vi "New Focus - rétroaction.vi"() -> ()   [LabVIEW 2017]
uses:
  dll/CmdLib.dll
  Type Def/Data cluster.ctl
panel:
  in  "Wavelength (nm)":u32=1064
  in  "Pas":i32=10
  in  "angle du max":i32=4500
  in  "ParameterPhi":dbl=38.36882237534376
  in  "ParameterC":dbl=2.6797703442087277
  in  "ParameterB":dbl=1.035346678618637e-36
  in  "ParameterA":dbl=0.997938844220231
  out "nombre":dbl
  out "DAQ?":bool
  in  "Mode":bool
  in  "VISA Refnum in":refnum<visa-resource-name>
  in  "consigne":dbl=23.0 format="%#_13g"
  in  "erreur en %":dbl(knob)=2.0 scale=0.0..10.0
  in  "Bouton Piste suivante":bool
  in  "Bouton Recherche en avant":bool
  in  "Bouton Recherche en arrière":bool
  in  "Bouton Piste précédente":bool
  out "tampon":i32=50
  out "Taux transmission calculé":dbl
  in  "Taux Transmission":dbl(knob)=0.98 min=0.02 max=0.98 scale=0.0..1.0
  in  "Maximum?":bool
  in  "Relative Steps":i32=50
  out "sortie d'erreur":errorcluster
  in  "Motor 3":bool
  in  "Motor 2":bool
  in  "Motor 1":bool
  in  "Bouton Stop":bool
  out "DeviceKey List Out":string[](array[string])
  out "error IO":errorcluster
  out "error out":errorcluster
  out "Device Array":T1(array[cluster])
  out "CmdLib Out":refnum<k24>
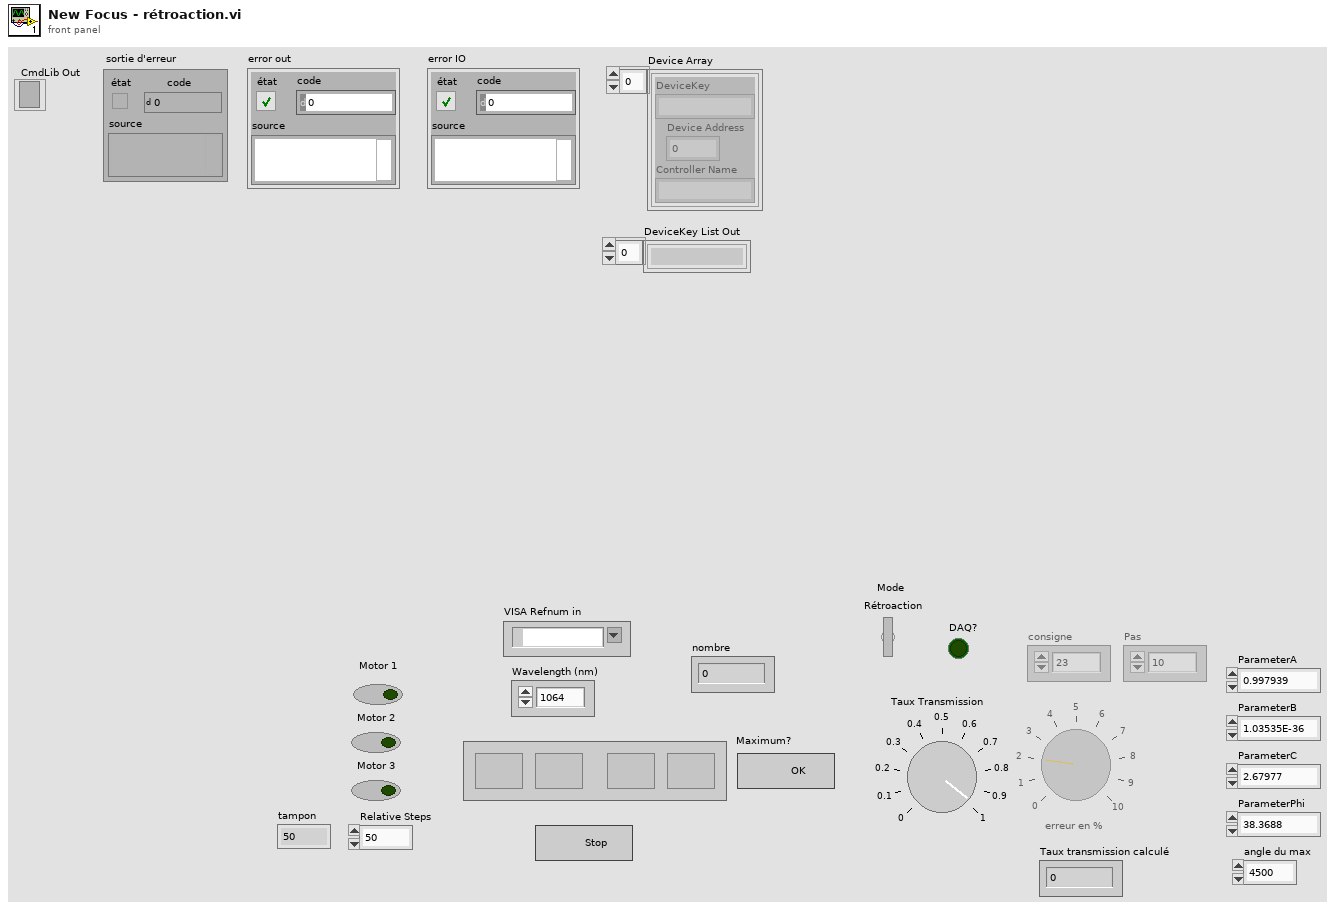
[diagram p1: front panel]
types:
  T1 = cluster{"DeviceKey":string, "Device Address":i32, "Controller Name":string}[]
  T2 = enum8{"Enabled", "Disabled", "Disabled and Grayed Out"}
  T3 = typedef "Data cluster.ctl" = cluster{enum16{"Init", "Control", "Stop"}, "Device Adress":i32, "Motor":i32, "Device Key":string, "Relative Steps":i32}
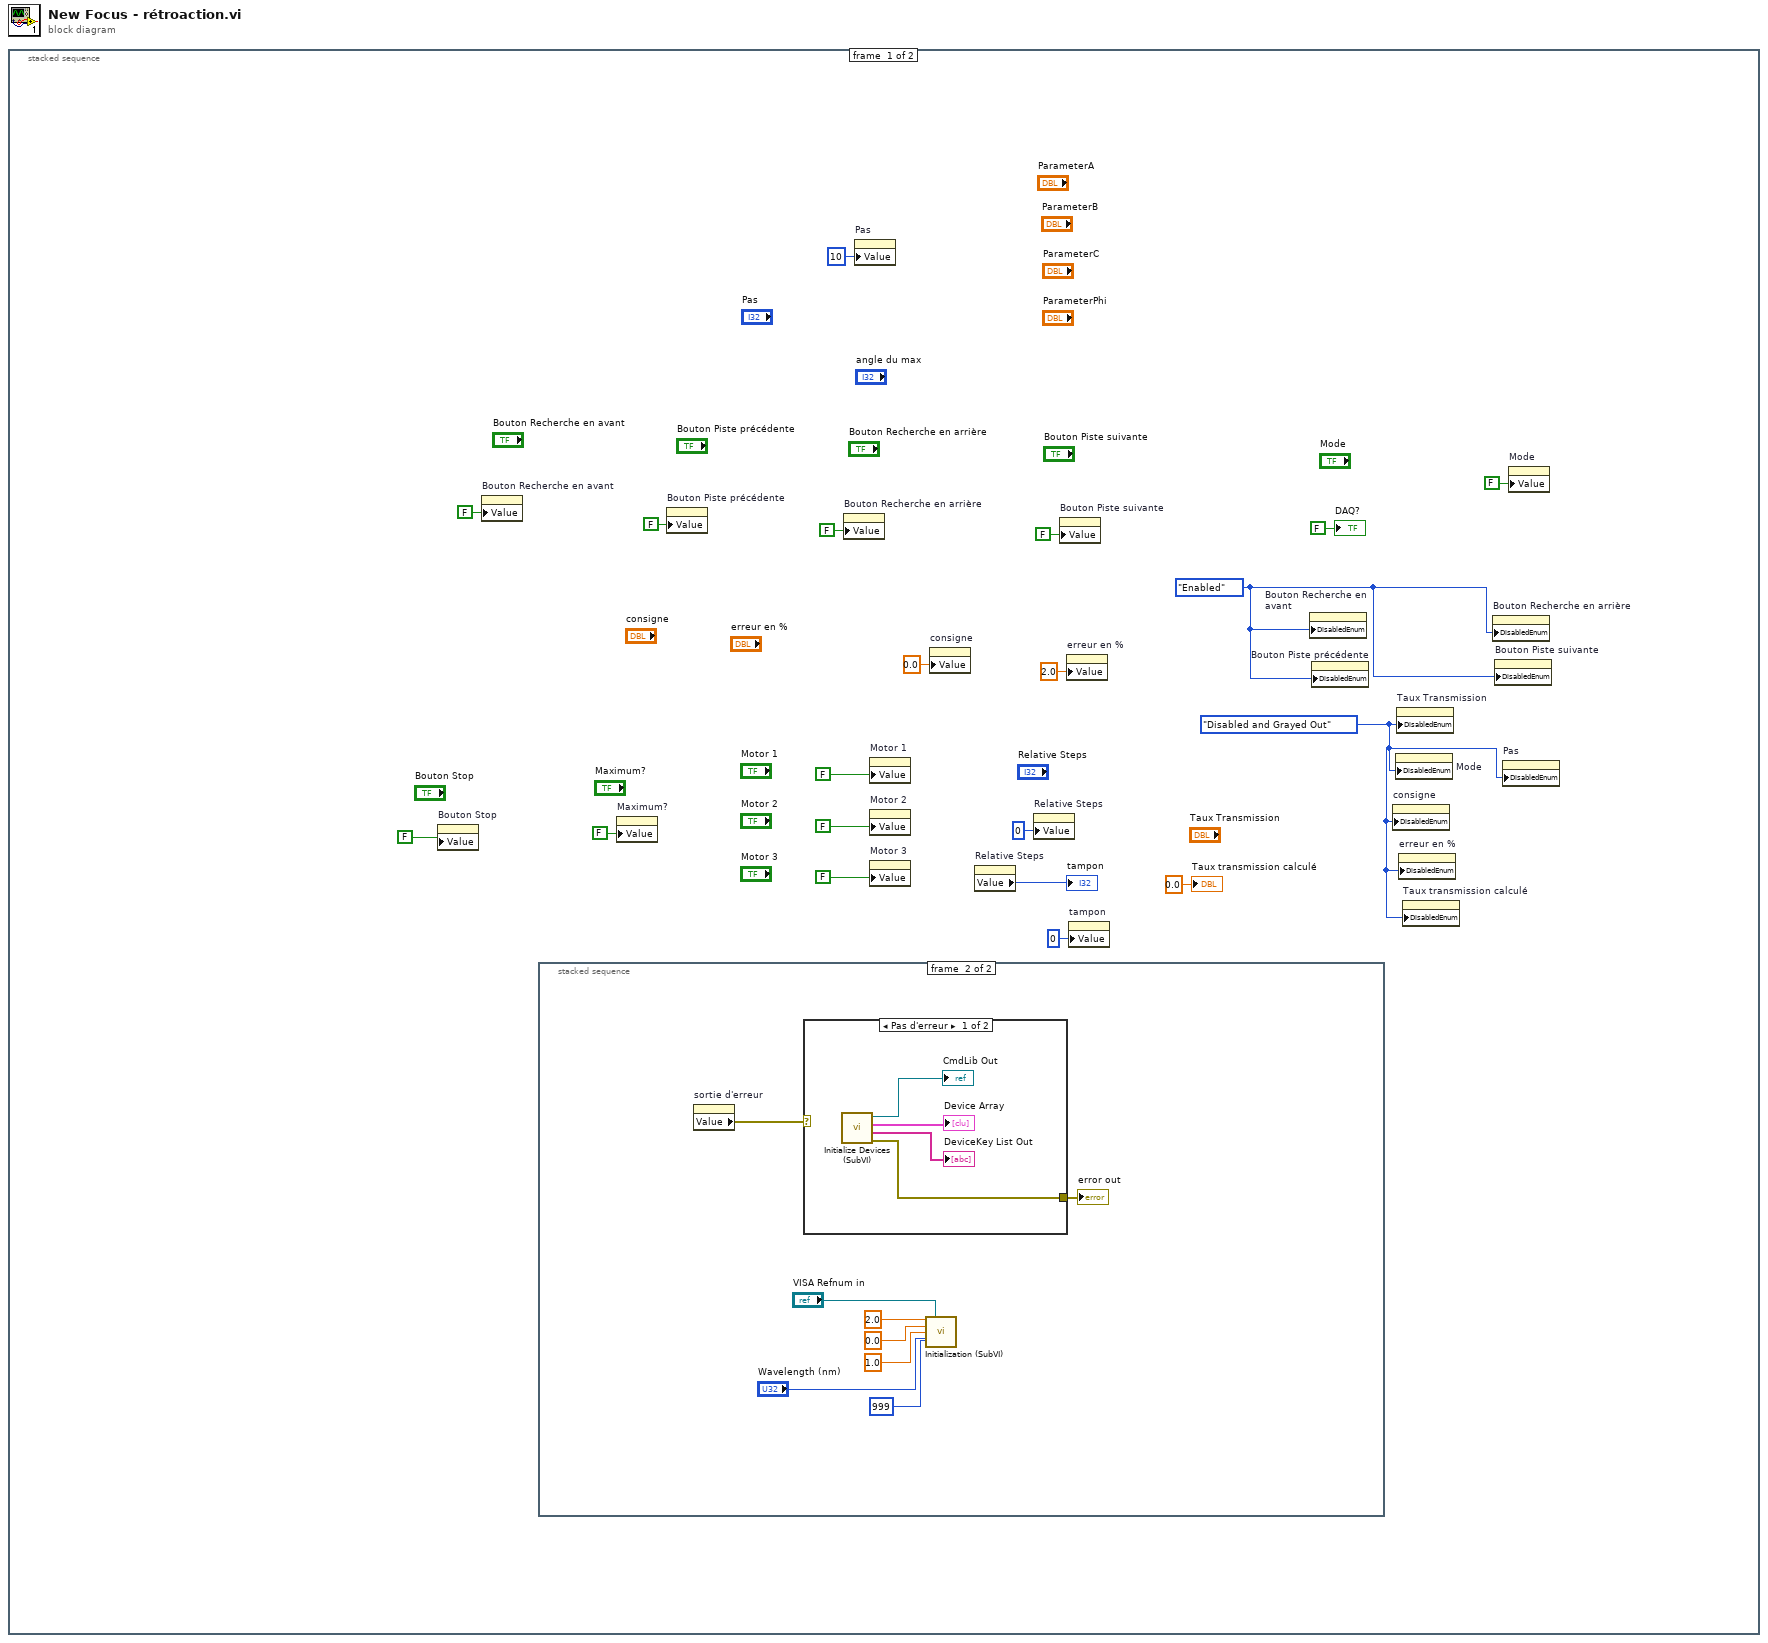
[diagram p0: block diagram]
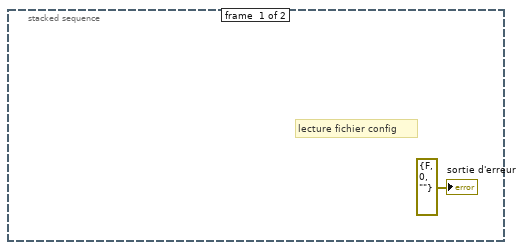
[diagram p2: hidden frame]
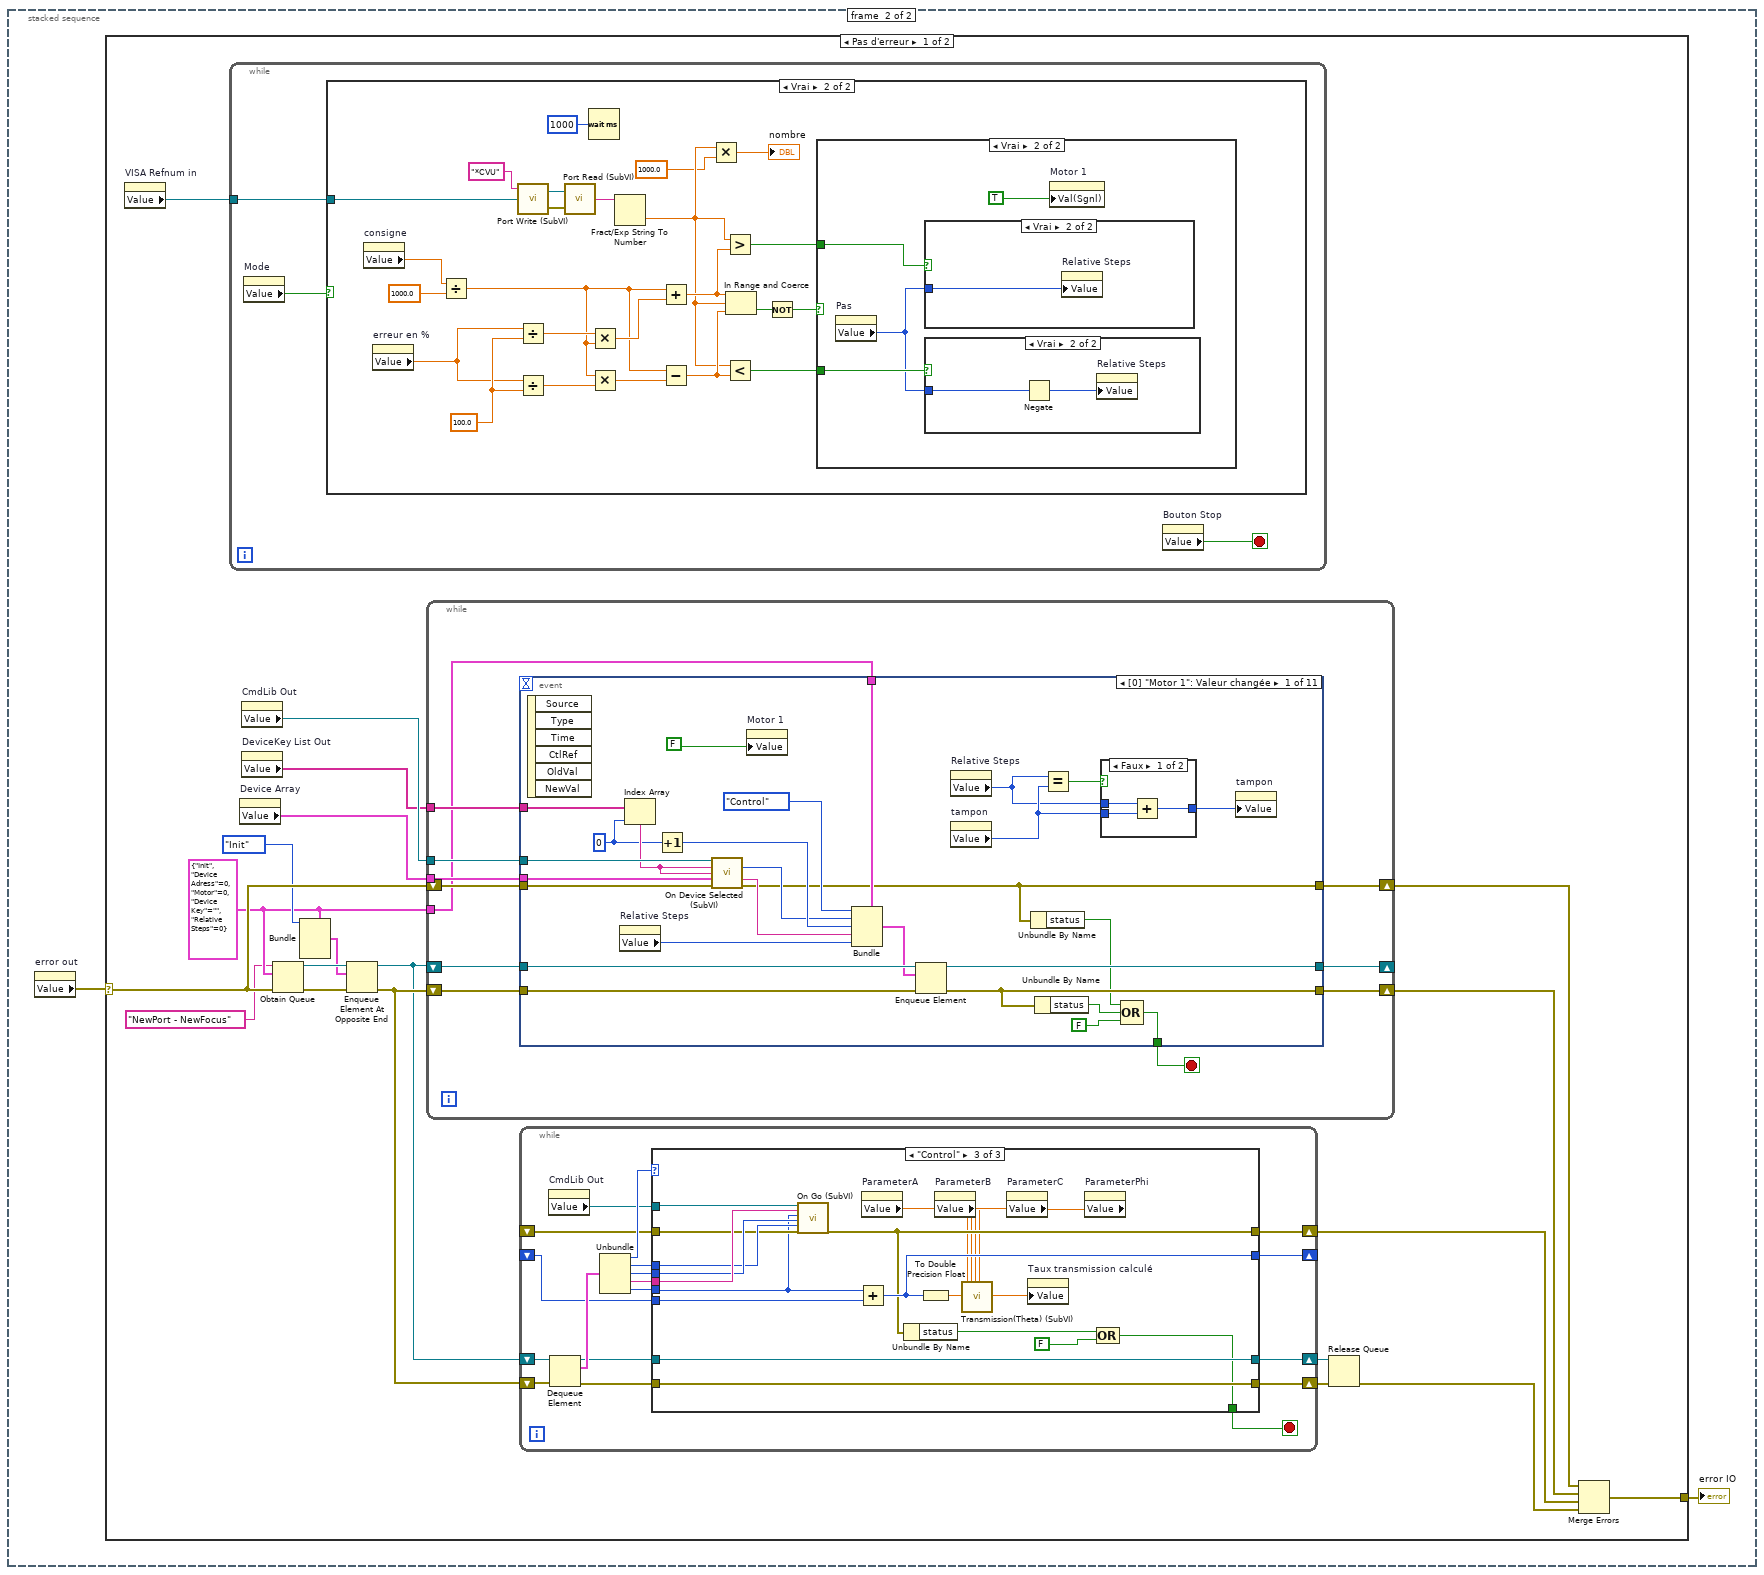
[diagram p4: hidden frame]
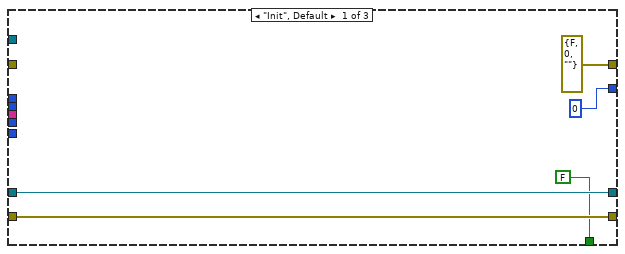
[diagram p9: hidden frame]
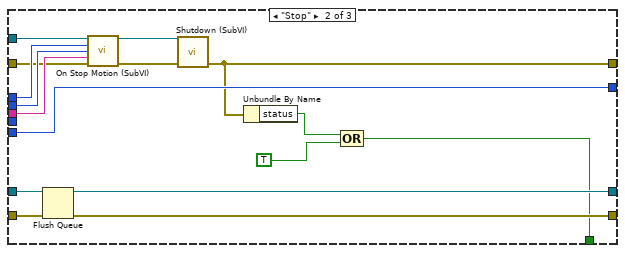
[diagram p10: hidden frame]
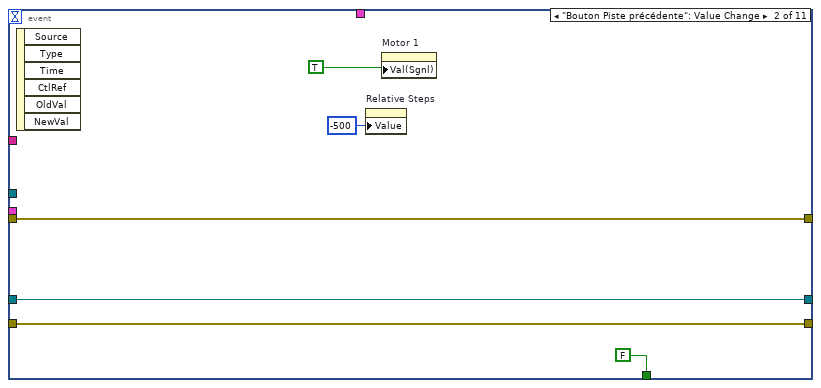
[diagram p12: hidden frame]
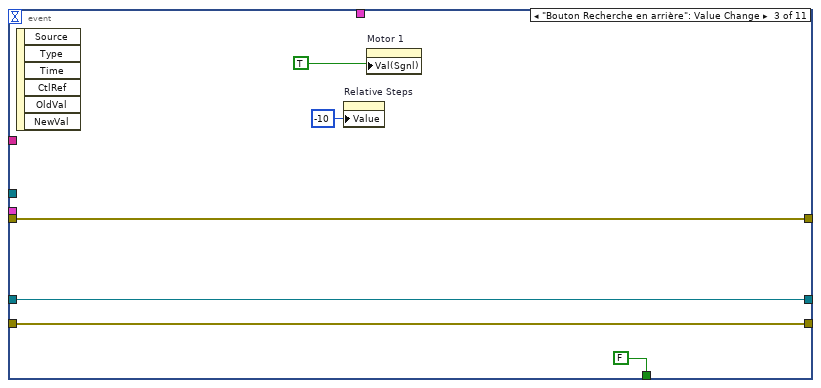
[diagram p13: hidden frame]
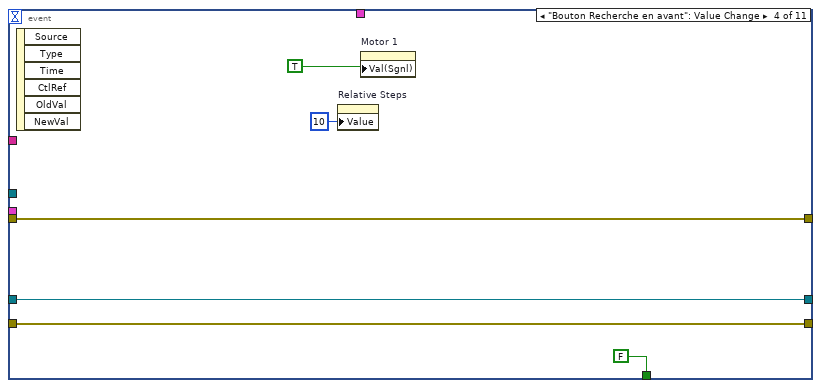
[diagram p14: hidden frame]
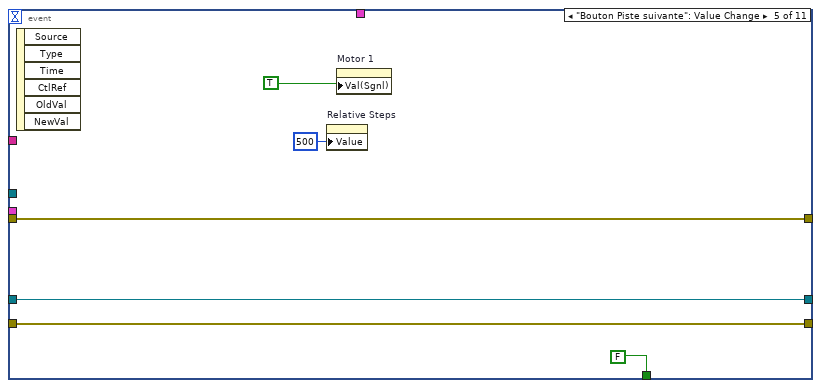
[diagram p15: hidden frame]
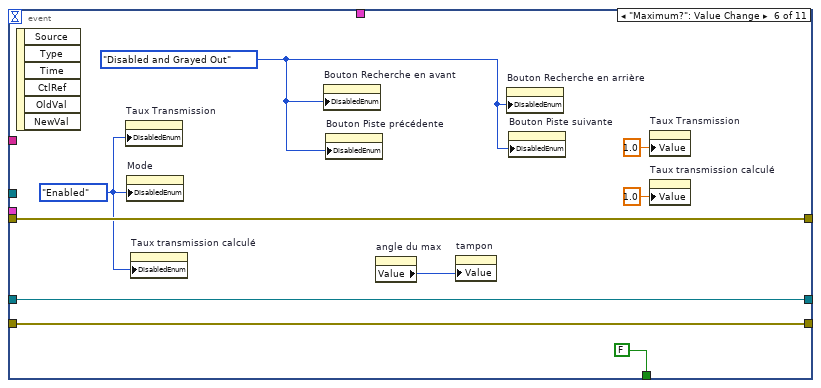
[diagram p16: hidden frame]
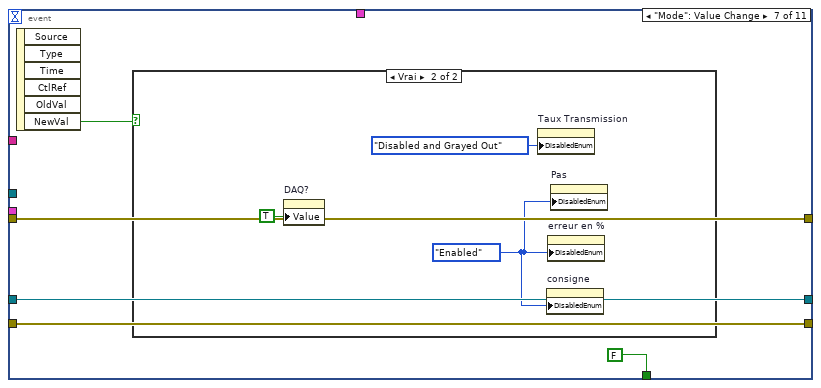
[diagram p17: hidden frame]
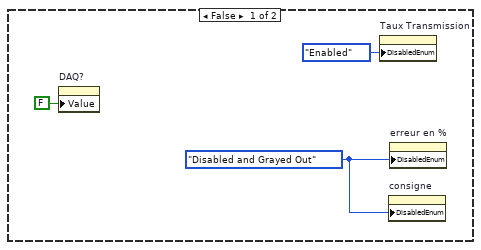
[diagram p18: hidden frame]
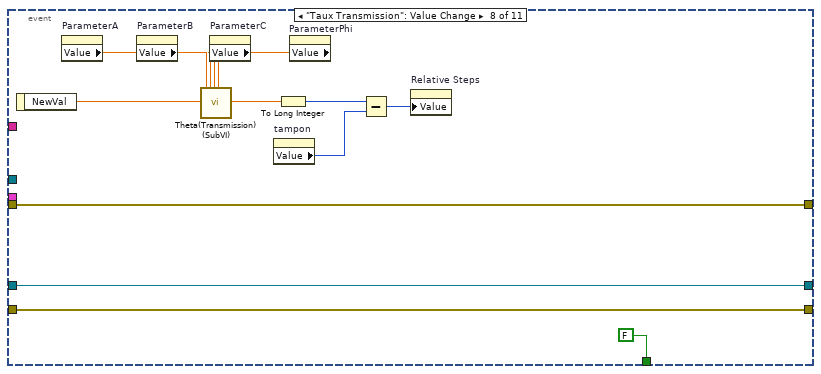
[diagram p19: hidden frame]
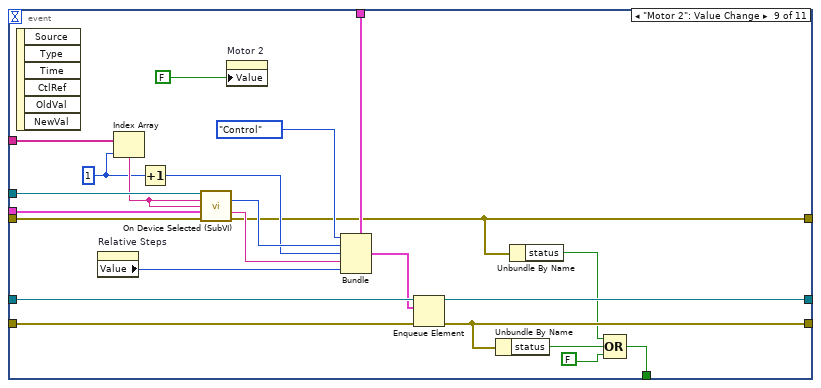
[diagram p20: hidden frame]
diagram:
  n1 = stacked-sequence {
    frame #0 {
      w2 = T2."Disabled and Grayed Out" ("Désactivé")
      w8 = T2."Enabled" ("Désactivé")
      n2 = property on="Bouton Stop" class="Bool (strict)"("Value"=FALSE) -> ()  [unwired: 2 in, 2 out]
      n3 = property on="Bouton Recherche en avant" class="Bool (strict)"("Value"=FALSE ("Bouton Recherche en avant")) -> ()  [unwired: 2 in, 2 out]
      n4 = stacked-sequence {
        frame #0 {
          # "lecture fichier config"
          "sortie d'erreur" <- errorcluster {"status"=FALSE, "code"=0, "source"=""} ("sortie d'erreur")
        }
        frame #1 {
          n5 = property on="sortie d'erreur" class="Clust (strict)"() -> ("Value"=w28:errorcluster)  [unwired: 2 in, 2 out]
          n6 = case shown="Pas d'erreur" w28 {
            selector: w28 -> [_ w34]
            tunnel: [w33 w34] -> w29
            frame No Error {
              n7 = call "Initialize Devices (SubVI).vi"() -> ("sortie d'erreur"=w33:errorcluster, "DeviceKey List Out"=→"DeviceKey List Out":string[], "Device Array"=→"Device Array":T1, "Refnum de .NET en sortie"=→"CmdLib Out":refnum<k24>)  [unwired: 8 in]
            }
            frame Error {
            }
          }
          "error out" <- w29
          n8 = call "Initialization (SubVI).vi"("Trigger Level (% of Scale)"=2.0, "VISA Refnum in"="VISA Refnum in", "Offset"=sgl 0.0, "Multiplier"=sgl 1.0, "Wavelength (nm)"="Wavelength (nm)", "Scale"=u32 999) -> ()  [unwired: 8 in, 2 out]
        }
      }
      n9 = property on="Maximum?" class="Bool (strict)"("Value"=FALSE ("Minimum?")) -> ()  [unwired: 2 in, 2 out]
      n10 = property on="Bouton Piste précédente" class="Bool (strict)"("Value"=FALSE ("Bouton Piste précédente")) -> ()  [unwired: 2 in, 2 out]
      n11 = property on="Bouton Recherche en arrière" class="Bool (strict)"("Value"=FALSE ("Bouton Recherche en arrière")) -> ()  [unwired: 2 in, 2 out]
      n12 = property on="Pas" class="NumNb (strict)"("Value"=10 ("Numérique")) -> ()  [unwired: 2 in, 2 out]
      n13 = property on="Motor 1" class="Bool (strict)"("Value"=FALSE) -> ()  [unwired: 2 in, 2 out]
      n14 = property on="Motor 2" class="Bool (strict)"("Value"=FALSE) -> ()  [unwired: 2 in, 2 out]
      n15 = property on="Motor 3" class="Bool (strict)"("Value"=FALSE) -> ()  [unwired: 2 in, 2 out]
      n16 = property on="consigne" class="NumNb (strict)"("Value"=0.0 ("consigne")) -> ()  [unwired: 2 in, 2 out]
      n17 = property on="Relative Steps" class="NumNb (strict)"() -> ("Value"=→"tampon":i32)  [unwired: 2 in, 2 out]
      n18 = property on="Relative Steps" class="NumNb (strict)"("Value"=0 ("Relative Steps")) -> ()  [unwired: 2 in, 2 out]
      n19 = property on="Bouton Piste suivante" class="Bool (strict)"("Value"=FALSE ("Bouton Piste suivante")) -> ()  [unwired: 2 in, 2 out]
      n20 = property on="erreur en %" class="BoutRot (strict)"("Value"=2.0 ("erreur en %")) -> ()  [unwired: 2 in, 2 out]
      n21 = property on="tampon" class="NumNb (strict)"("Value"=0 ("tampon")) -> ()  [unwired: 2 in, 2 out]
      n22 = property on="Bouton Recherche en avant" class="Bool (strict)"("DisabledEnum"=w8) -> ()  [unwired: 2 in, 2 out]
      n23 = property on="Bouton Piste précédente" class="Bool (strict)"("DisabledEnum"=w8) -> ()  [unwired: 2 in, 2 out]
      n24 = property on="consigne" class="NumNb (strict)"("DisabledEnum"=w2) -> ()  [unwired: 2 in, 2 out]
      n25 = property on="Mode" class="Bool (strict)"("DisabledEnum"=w2) -> ()  [unwired: 2 in, 2 out]
      n26 = property on="Taux Transmission" class="BoutRot (strict)"("DisabledEnum"=w2) -> ()  [unwired: 2 in, 2 out]
      n27 = property on="erreur en %" class="BoutRot (strict)"("DisabledEnum"=w2) -> ()  [unwired: 2 in, 2 out]
      n28 = property on="Taux transmission calculé" class="NumNb (strict)"("DisabledEnum"=w2) -> ()  [unwired: 2 in, 2 out]
      n29 = property on="Bouton Recherche en arrière" class="Bool (strict)"("DisabledEnum"=w8) -> ()  [unwired: 2 in, 2 out]
      n30 = property on="Bouton Piste suivante" class="Bool (strict)"("DisabledEnum"=w8) -> ()  [unwired: 2 in, 2 out]
      n31 = property on="Pas" class="NumNb (strict)"("DisabledEnum"=w2) -> ()  [unwired: 2 in, 2 out]
      n32 = property on="Mode" class="Bool (strict)"("Value"=FALSE ("Mode")) -> ()  [unwired: 2 in, 2 out]
      "Taux transmission calculé" <- 0.0 ("x-y")
      "DAQ?" <- FALSE ("DAQ?")
    }
    frame #1 {
      n33 = property on="error out" class="Clust (strict)"() -> ("Value"=w36:errorcluster)  [unwired: 2 in, 2 out]
      n34 = case shown="Pas d'erreur" w36 {
        selector: w36 -> [w55 w327]
        tunnel: [w56 w327] -> w35
        frame No Error {
          w48 = T3 {enum."Init", "Device Adress"=0, "Motor"=0, "Device Key"="", "Relative Steps"=0}
          n35 = property on="VISA Refnum in" class="NomVISA"() -> ("Value"=w37:refnum<visa-resource-name>)  [unwired: 2 in, 2 out]
          n36 = while {
            tunnel: w37 -> [w57]
            stop <- w59 stop-if-true
            n37 = property on="Mode" class="Bool (strict)"() -> ("Value"=w58:bool)  [unwired: 2 in, 2 out]
            n38 = case shown="Vrai" w58 {
              tunnel: w57 -> [_ w66]
              frame False {
              }
              frame True {
                w74 = 100.0 ("y")
                n39 = property on="consigne" class="NumNb (strict)"() -> ("Value"=w61:dbl)  [unwired: 2 in, 2 out]
                n40 = property on="erreur en %" class="BoutRot (strict)"() -> ("Value"=w71:dbl)  [unwired: 2 in, 2 out]
                n41 = Divide(x=w61, y=1000.0) -> (x/y=w62:dbl)
                n42 = call "Port Write (SubVI).vi"("VISA Refnum in"=w66, "write buffer"="*CVU") -> ("error out"=w80:errorcluster, "VISA Refnum out"=w81:refnum<visa-resource-name>)  [unwired: 1 in]
                n43 = Divide(x=w71, y=w74) -> (x/y=w78:dbl)
                n44 = Divide(x=w71, y=w74) -> (x/y=w75:dbl)
                n45 = call "Port Read (SubVI).vi"("VISA Refnum in"=w81, "error in"=w80) -> ("buffer read"=w79:string)  [unwired: 2 out]
                n46 = Wait (ms)(milliseconds to wait=u32 1000 ("attente (ms)")) -> ()  [unwired: 1 out]
                n47 = Multiply(x=w78, y=w62) -> (x*y=w76:dbl)
                n48 = Multiply(x=w62, y=w75) -> (x*y=w77:dbl)
                n49 = Fract/Exp String To Number(string=w79) -> (number=w64:dbl)  [unwired: 3 in, 1 out]
                n50 = Add(x=w62, y=w76) -> (x+y=w73:dbl)
                n51 = Subtract(x=w62, y=w77) -> (x-y=w72:dbl)
                n52 = Multiply(x=w64, y=1000.0) -> (x*y=→"nombre":dbl)
                n53 = Greater?(x=w64, y=w73) -> (0:w69:bool)
                n54 = Less?(x=w64, y=w72) -> (x < y?=w70:bool)
                n55 = In Range and Coerce(upper limit=w73, x=w64, lower limit=w72) -> (In Range?=w68:bool)  [unwired: 1 out]
                n56 = Not(x=w68) -> (.not. x?=w67:bool)
                n57 = case shown="Vrai" w67 {
                  tunnel: w70 -> [_ w86]
                  tunnel: w69 -> [_ w85]
                  frame False {
                  }
                  frame True {
                    n58 = property on="Pas" class="NumNb (strict)"() -> ("Value"=w84:i32)  [unwired: 2 in, 2 out]
                    n59 = case shown="Vrai" w85 {
                      tunnel: w84 -> [_ w90]
                      frame False {
                      }
                      frame True {
                        n60 = property on="Relative Steps" class="NumNb (strict)"("Value"=w90) -> ()  [unwired: 2 in, 2 out]
                      }
                    }
                    n61 = case shown="Vrai" w86 {
                      tunnel: w84 -> [_ w88]
                      frame False {
                      }
                      frame True {
                        n62 = Negate(x=w88) -> (-x=w89:i32)
                        n63 = property on="Relative Steps" class="NumNb (strict)"("Value"=w89) -> ()  [unwired: 2 in, 2 out]
                      }
                    }
                    n64 = property on="Motor 1" class="Bool (strict)"("Val(Sgnl)"=TRUE ("Valeur (Signalisation)")) -> ()  [unwired: 2 in, 2 out]
                  }
                }
              }
            }
            n65 = property on="Bouton Stop" class="Bool (strict)"() -> ("Value"=w59:bool)  [unwired: 2 in, 2 out]
          }
          n66 = property on="Device Array" class="Tabl (strict)"() -> ("Value"=w46:T1)  [unwired: 2 in, 2 out]
          n67 = property on="CmdLib Out" class="Ref (strict)"() -> ("Value"=w47:refnum<k24>)  [unwired: 2 in, 2 out]
          n68 = property on="DeviceKey List Out" class="Tabl (strict)"() -> ("Value"=w40:string[])  [unwired: 2 in, 2 out]
          n69 = Obtain Queue(name (unnamed)="NewPort - NewFocus" ("nom (aucun)"), element data type=w48, error in (no error)=w55) -> (queue out=w53:refnum<queue>, error out=w54:errorcluster)  [unwired: 2 in, 1 out]
          n70 = Bundle(cluster=w48, enum16{"Init", "Control", "Stop"}."Init") -> (w51:T3)  [unwired: 4 in]
          n71 = Enqueue Element At Opposite End(queue=w53, element=w51, error in (no error)=w54) -> (queue out=w49:refnum<queue>, error out=w50:errorcluster)  [unwired: 1 in, 1 out]
          n72 = while {
            shift-right: [w150] -> w42
            shift-left: w50 -> [w160]
            shift-right: [w151] -> _
            shift-left: w49 -> [w159]
            tunnel: w48 -> [w152]
            tunnel: w47 -> [w158]
            tunnel: w46 -> [w157]
            shift-right: [w156] -> w41
            shift-left: w55 -> [w155]
            tunnel: w40 -> [w153]
            stop <- w154 stop-if-true
            n73 = event shown="[0] \"Motor 1\": Valeur changée" {
              selector: _ -> [_ _ _ _ _ _ _ _ _ _ _]
              dyn-events: _ -> [_ _ _ _ _ _ _ _ _ _ _]
              timeout: _ -> [_ _ _ _ _ _ _ _ _ _ _]
              tunnel: w160 -> [w173 w193 w199 w205 w212 w221 w228 w246 w262 w279 w306]
              tunnel: [w165 w193 w199 w205 w212 w221 w228 w246 w253 w277 w300] -> w150
              tunnel: w159 -> [w174 w194 w200 w206 w213 w222 w229 w247 w263 w281 w307]
              tunnel: [w175 w194 w200 w206 w213 w222 w229 w247 w261 w280 w305] -> w151
              tunnel: w158 -> [w187 _ _ _ _ _ _ _ w271 w294 w309]
              tunnel: w157 -> [w183 _ _ _ _ _ _ _ w268 w291 w303]
              tunnel: [w166 w195 w201 w207 w211 w223 w227 w245 w254 w276 w299] -> w156
              tunnel: w155 -> [w186 w195 w201 w207 w211 w223 w227 w245 w270 w293 w308]
              tunnel: [w161 FALSE FALSE FALSE FALSE FALSE FALSE FALSE w249 w275 w298] -> w154
              tunnel: w153 -> [w184 _ _ _ _ _ _ _ w269 w292 w302]
              tunnel: w152 -> [w180 _ _ _ _ _ _ _ w264 w287 w301]
              event "Motor 1": Value Change {
                w181 = 0
                n74 = event-data() -> ()  [unwired: 1 in, 6 out]
                n75 = property on="Relative Steps" class="NumNb (strict)"() -> ("Value"=w171:i32)  [unwired: 2 in, 2 out]
                n76 = Index Array(array=w184, index=w181) -> (element=w182:string)
                n77 = Increment(x=w181) -> (x+1=w178:i32)
                n78 = call "On Device Selected (SubVI).vi"("CmdLib In"=w187, "Device Key"=w182, "Device Key In"=w182, "Device Array"=w183, "error in"=w186) -> ("Device Address"=w177:i32, "Device Key Out"=w179:string, "error out"=w166:errorcluster)  [unwired: 8 in]
                n79 = property on="Motor 1" class="Bool (strict)"("Value"=FALSE) -> ()  [unwired: 2 in, 2 out]
                n80 = Bundle(cluster=w180, enum16{"Init", "Control", "Stop"}."Control", "Device Adress"=w177, "Motor"=w178, "Device Key"=w179, "Relative Steps"=w171) -> (w172:T3)
                n81 = Enqueue Element(queue=w174, element=w172, error in (no error)=w173) -> (queue out=w175:refnum<queue>, error out=w165:errorcluster)  [unwired: 1 in, 1 out]
                n82 = property on="Relative Steps" class="NumNb (strict)"() -> ("Value"=w168:i32)  [unwired: 2 in, 2 out]
                n83 = property on="tampon" class="NumNb (strict)"() -> ("Value"=w169:i32)  [unwired: 2 in, 2 out]
                n84 = Unbundle By Name(w166) -> ("status"=w162:bool)
                n85 = Unbundle By Name(w165) -> ("status"=w163:bool)
                n86 = Equal?(x=w168, y=w169) -> (x = y?=w167:bool)
                n87 = case shown="Faux" w167 {
                  tunnel: [w190 w191] -> w170
                  tunnel: w169 -> [w189 _]
                  tunnel: w168 -> [w188 w191]
                  frame False {
                    n88 = Add(x=w188, y=w189) -> (x+y=w190:i32)
                  }
                  frame True {
                  }
                }
                n89 = Compound Arithmetic op=OR ("Opérateur arithmétique")(w162, w163, FALSE) -> (w161:bool)
                n90 = property on="tampon" class="NumNb (strict)"("Value"=w170) -> ()  [unwired: 2 in, 2 out]
              }
              event "Bouton Piste précédente": Value Change {
                n91 = event-data() -> ()  [unwired: 1 in, 6 out]
                n92 = property on="Relative Steps" class="NumNb (strict)"("Value"=-500 ("Relative Steps")) -> ()  [unwired: 2 in, 2 out]
                n93 = property on="Motor 1" class="Bool (strict)"("Val(Sgnl)"=TRUE) -> ()  [unwired: 2 in, 2 out]
              }
              event "Bouton Recherche en arrière": Value Change {
                n94 = event-data() -> ()  [unwired: 1 in, 6 out]
                n95 = property on="Relative Steps" class="NumNb (strict)"("Value"=-10 ("Relative Steps")) -> ()  [unwired: 2 in, 2 out]
                n96 = property on="Motor 1" class="Bool (strict)"("Val(Sgnl)"=TRUE) -> ()  [unwired: 2 in, 2 out]
              }
              event "Bouton Recherche en avant": Value Change {
                n97 = event-data() -> ()  [unwired: 1 in, 6 out]
                n98 = property on="Relative Steps" class="NumNb (strict)"("Value"=10 ("Relative Steps")) -> ()  [unwired: 2 in, 2 out]
                n99 = property on="Motor 1" class="Bool (strict)"("Val(Sgnl)"=TRUE) -> ()  [unwired: 2 in, 2 out]
              }
              event "Bouton Piste suivante": Value Change {
                n100 = event-data() -> ()  [unwired: 1 in, 6 out]
                n101 = property on="Relative Steps" class="NumNb (strict)"("Value"=500 ("Relative Steps")) -> ()  [unwired: 2 in, 2 out]
                n102 = property on="Motor 1" class="Bool (strict)"("Val(Sgnl)"=TRUE) -> ()  [unwired: 2 in, 2 out]
              }
              event "Maximum?": Value Change {
                w217 = T2."Enabled" ("Désactivé")
                w220 = T2."Disabled and Grayed Out" ("Désactivé")
                n103 = event-data() -> ()  [unwired: 1 in, 6 out]
                n104 = property on="Taux Transmission" class="BoutRot (strict)"("DisabledEnum"=w217) -> ()  [unwired: 2 in, 2 out]
                n105 = property on="Mode" class="Bool (strict)"("DisabledEnum"=w217) -> ()  [unwired: 2 in, 2 out]
                n106 = property on="Taux transmission calculé" class="NumNb (strict)"("DisabledEnum"=w217) -> ()  [unwired: 2 in, 2 out]
                n107 = property on="Bouton Recherche en avant" class="Bool (strict)"("DisabledEnum"=w220) -> ()  [unwired: 2 in, 2 out]
                n108 = property on="Bouton Piste précédente" class="Bool (strict)"("DisabledEnum"=w220) -> ()  [unwired: 2 in, 2 out]
                n109 = property on="angle du max" class="NumNb (strict)"() -> ("Value"=w216:i32)  [unwired: 2 in, 2 out]
                n110 = property on="tampon" class="NumNb (strict)"("Value"=w216) -> ()  [unwired: 2 in, 2 out]
                n111 = property on="Bouton Recherche en arrière" class="Bool (strict)"("DisabledEnum"=w220) -> ()  [unwired: 2 in, 2 out]
                n112 = property on="Bouton Piste suivante" class="Bool (strict)"("DisabledEnum"=w220) -> ()  [unwired: 2 in, 2 out]
                n113 = property on="Taux Transmission" class="BoutRot (strict)"("Value"=1.0 ("Glissière")) -> ()  [unwired: 2 in, 2 out]
                n114 = property on="Taux transmission calculé" class="NumNb (strict)"("Value"=1.0 ("Taux transmission calculé")) -> ()  [unwired: 2 in, 2 out]
              }
              event "Mode": Value Change {
                n115 = event-data() -> ("NewVal"=w226:bool)  [unwired: 1 in, 5 out]
                n116 = case shown="Vrai" w226 {
                  frame False {
                    w232 = T2."Disabled and Grayed Out" ("Désactivé")
                    n117 = property on="DAQ?" class="Bool (strict)"("Value"=FALSE ("DAQ?")) -> ()  [unwired: 2 in, 2 out]
                    n118 = property on="Taux Transmission" class="BoutRot (strict)"("DisabledEnum"=T2."Enabled" ("Désactivé")) -> ()  [unwired: 2 in, 2 out]
                    n119 = property on="consigne" class="NumNb (strict)"("DisabledEnum"=w232) -> ()  [unwired: 2 in, 2 out]
                    n120 = property on="erreur en %" class="BoutRot (strict)"("DisabledEnum"=w232) -> ()  [unwired: 2 in, 2 out]
                  }
                  frame True {
                    w233 = T2."Enabled" ("Désactivé")
                    n121 = property on="DAQ?" class="Bool (strict)"("Value"=TRUE ("DAQ?")) -> ()  [unwired: 2 in, 2 out]
                    n122 = property on="Taux Transmission" class="BoutRot (strict)"("DisabledEnum"=T2."Disabled and Grayed Out" ("Désactivé")) -> ()  [unwired: 2 in, 2 out]
                    n123 = property on="consigne" class="NumNb (strict)"("DisabledEnum"=w233) -> ()  [unwired: 2 in, 2 out]
                    n124 = property on="erreur en %" class="BoutRot (strict)"("DisabledEnum"=w233) -> ()  [unwired: 2 in, 2 out]
                    n125 = property on="Pas" class="NumNb (strict)"("DisabledEnum"=w233) -> ()  [unwired: 2 in, 2 out]
                  }
                }
              }
              event "Taux Transmission": Value Change {
                n126 = event-data() -> ("NewVal"=w243:dbl)  [unwired: 1 in]
                n127 = property on="ParameterA" class="NumNb (strict)"() -> ("Value"=w239:dbl)  [unwired: 2 in, 2 out]
                n128 = property on="ParameterB" class="NumNb (strict)"() -> ("Value"=w238:dbl)  [unwired: 2 in, 2 out]
                n129 = property on="ParameterC" class="NumNb (strict)"() -> ("Value"=w237:dbl)  [unwired: 2 in, 2 out]
                n130 = property on="tampon" class="NumNb (strict)"() -> ("Value"=w241:i32)  [unwired: 2 in, 2 out]
                n131 = property on="ParameterPhi" class="NumNb (strict)"() -> ("Value"=w236:dbl)  [unwired: 2 in, 2 out]
                n132 = call "Theta(Transmission) (SubVI).vi"("Transmission"=w243, "ParameterA"=w239, "ParameterB"=w238, "ParameterC"=w237, "ParameterPhi"=w236) -> ("Position_calcul"=w242:dbl)  [unwired: 22 in]
                n133 = To Long Integer(number=w242) -> (32bit integer=w240:i32)
                n134 = Subtract(x=w240, y=w241) -> (x-y=w244:i32)
                n135 = property on="Relative Steps" class="NumNb (strict)"("Value"=w244) -> ()  [unwired: 2 in, 2 out]
              }
              event "Motor 2": Value Change {
                w266 = 1
                n136 = event-data() -> ()  [unwired: 1 in, 6 out]
                n137 = property on="Relative Steps" class="NumNb (strict)"() -> ("Value"=w260:i32)  [unwired: 2 in, 2 out]
                n138 = Index Array(array=w269, index=w266) -> (element=w267:string)
                n139 = Increment(x=w266) -> (x+1=w257:i32)
                n140 = call "On Device Selected (SubVI).vi"("CmdLib In"=w271, "Device Key"=w267, "Device Key In"=w267, "Device Array"=w268, "error in"=w270) -> ("Device Address"=w258:i32, "Device Key Out"=w259:string, "error out"=w254:errorcluster)  [unwired: 8 in]
                n141 = property on="Motor 2" class="Bool (strict)"("Value"=FALSE) -> ()  [unwired: 2 in, 2 out]
                n142 = Bundle(cluster=w264, enum16{"Init", "Control", "Stop"}."Control", "Device Adress"=w258, "Motor"=w257, "Device Key"=w259, "Relative Steps"=w260) -> (w255:T3)
                n143 = Enqueue Element(queue=w263, element=w255, error in (no error)=w262) -> (queue out=w261:refnum<queue>, error out=w253:errorcluster)  [unwired: 1 in, 1 out]
                n144 = Unbundle By Name(w253) -> ("status"=w251:bool)
                n145 = Unbundle By Name(w254) -> ("status"=w252:bool)
                n146 = Compound Arithmetic op=OR ("Opérateur arithmétique")(w252, w251, FALSE) -> (w249:bool)
              }
              event "Motor 3": Value Change {
                w289 = 2
                n147 = event-data() -> ()  [unwired: 1 in, 6 out]
                n148 = Index Array(array=w292, index=w289) -> (element=w290:string)
                n149 = property on="Relative Steps" class="NumNb (strict)"() -> ("Value"=w286:i32)  [unwired: 2 in, 2 out]
                n150 = call "On Device Selected (SubVI).vi"("CmdLib In"=w294, "Device Key"=w290, "Device Key In"=w290, "Device Array"=w291, "error in"=w293) -> ("Device Address"=w283:i32, "Device Key Out"=w285:string, "error out"=w276:errorcluster)  [unwired: 8 in]
                n151 = Increment(x=w289) -> (x+1=w284:i32)
                n152 = property on="Motor 3" class="Bool (strict)"("Value"=FALSE) -> ()  [unwired: 2 in, 2 out]
                n153 = Bundle(cluster=w287, enum16{"Init", "Control", "Stop"}."Control", "Device Adress"=w283, "Motor"=w284, "Device Key"=w285, "Relative Steps"=w286) -> (w278:T3)
                n154 = Enqueue Element(queue=w281, element=w278, error in (no error)=w279) -> (queue out=w280:refnum<queue>, error out=w277:errorcluster)  [unwired: 1 in, 1 out]
                n155 = Unbundle By Name(w276) -> ("status"=w272:bool)
                n156 = Unbundle By Name(w277) -> ("status"=w273:bool)
                n157 = Compound Arithmetic op=OR ("Opérateur arithmétique")(w272, w273, FALSE) -> (w275:bool)
              }
              event "Bouton Stop": Value Change {
                n158 = event-data() -> ()  [unwired: 1 in, 1 out]
                n159 = Array Size(array=w303) -> (size(s)=w304:i32)
                n160 = for {
                  N: w304 -> [_]
                  tunnel: w309 -> [w323]
                  tunnel: w303 -> [w315]
                  tunnel: w308 -> [w322]
                  tunnel: [w317] -> w299
                  shift-right: [w318] -> w305
                  shift-left: w307 -> [w321]
                  shift-right: [w319] -> w300
                  shift-left: w306 -> [w320]
                  tunnel: w302 -> [w316]
                  tunnel: w301 -> [w311]
                  i -> [w313]
                  n161 = Index Array(array=w316, index=w313) -> (element=w314:string)
                  n162 = Increment(x=w313) -> (x+1=w310:i32)
                  n163 = call "On Device Selected (SubVI).vi"("CmdLib In"=w323, "Device Key"=w314, "Device Key In"=w314, "Device Array"=w315, "error in"=w322) -> ("Device Address"=w324:i32, "Device Key Out"=w326:string, "error out"=w317:errorcluster)  [unwired: 8 in]
                  n164 = Bundle(cluster=w311, enum16{"Init", "Control", "Stop"}."Stop", "Device Adress"=w324, "Motor"=w310, "Device Key"=w326) -> (w312:T3)  [unwired: 1 in]
                  n165 = Enqueue Element(queue=w321, element=w312, error in (no error)=w320) -> (queue out=w318:refnum<queue>, error out=w319:errorcluster)  [unwired: 1 in, 1 out]
                }
                n166 = Unbundle By Name(w299) -> ("status"=w295:bool)
                n167 = Unbundle By Name(w300) -> ("status"=w296:bool)
                n168 = Compound Arithmetic op=OR ("Opérateur arithmétique")(w295, w296, TRUE) -> (w298:bool)
              }
            }
          }
          n169 = while {
            shift-right: [w101] -> w45
            shift-left: w50 -> [w107]
            shift-right: [w100] -> w44
            shift-left: w49 -> [w108]
            shift-right: [w95] -> w39
            shift-left: _ -> [w94]
            shift-right: [w92] -> _
            shift-left: _ -> [w91]
            stop <- w96 stop-if-true
            n170 = property on="CmdLib Out" class="Ref (strict)"() -> ("Value"=w97:refnum<k24>)  [unwired: 2 in, 2 out]
            n171 = Dequeue Element(queue=w108, error in (no error)=w107) -> (queue out=w99:refnum<queue>, element=w106:T3, error out=w102:errorcluster)  [unwired: 1 in, 1 out]
            n172 = Unbundle(w106) -> (w105:enum16{"Init", "Control", "Stop"}, "Device Adress"=w104:i32, "Motor"=w103:i32, "Device Key"=w98:string, "Relative Steps"=w93:i32)
            n173 = case shown="\"Control\"" w105 {
              tunnel: w104 -> [_ w124 w144]
              tunnel: w103 -> [_ w122 w145]
              tunnel: w102 -> [w112 w129 w149]
              tunnel: [w112 w128 w149] -> w101
              tunnel: [w113 w127 w148] -> w100
              tunnel: w99 -> [w113 w126 w148]
              tunnel: w98 -> [_ w125 w146]
              tunnel: [errorcluster {"status"=FALSE, "code"=0, "source"=""} ("error out") w117 w138] -> w95
              tunnel: w97 -> [_ w123 w147]
              tunnel: [FALSE w114 w135] -> w96
              tunnel: w94 -> [_ w121 w143]
              tunnel: w93 -> [_ _ w139]
              tunnel: w91 -> [_ w118 w142]
              tunnel: [0 ("Relative Steps") w118 w140] -> w92
              frame "Init", Default {
              }
              frame "Stop" {
                n174 = Flush Queue(queue=w126, error in (no error)=w129) -> (queue out=w127:refnum<queue>, error out=w128:errorcluster)  [unwired: 1 out]
                n175 = call "On Stop Motion (SubVI).vi"("CmdLib In"=w123, "Device Address In"=w124, "Motor"=w122, "DeviceKey In"=w125, "error in"=w121) -> ("CmdLib In Out"=w119:refnum<k24>, "error out"=w120:errorcluster)  [unwired: 9 in]
                n176 = call "Shutdown (SubVI).vi"("error in (no error)"=w120, "CmdLib In"=w119) -> ("error out"=w117:errorcluster)  [unwired: 8 in, 1 out]
                n177 = Unbundle By Name(w117) -> ("status"=w116:bool)
                n178 = Compound Arithmetic op=OR ("Opérateur arithmétique")(w116, TRUE) -> (w114:bool)
              }
              frame "Control" {
                n179 = call "On Go (SubVI).vi"("CmdLib Out"=w147, "Device Key"=w146, "Relative Steps"=w139, "Motor"=w145, "Device Address"=w144, "error in"=w143) -> ("error out"=w138:errorcluster)  [unwired: 13 in]
                n180 = Add(x=w139, y=w142) -> (x+y=w140:i32)
                n181 = property on="ParameterA" class="NumNb (strict)"() -> ("Value"=w134:dbl)  [unwired: 2 in, 2 out]
                n182 = Unbundle By Name(w138) -> ("status"=w136:bool)
                n183 = To Double Precision Float(number=w140) -> (double precision float=w130:dbl)
                n184 = property on="ParameterB" class="NumNb (strict)"() -> ("Value"=w133:dbl)  [unwired: 2 in, 2 out]
                n185 = property on="ParameterC" class="NumNb (strict)"() -> ("Value"=w132:dbl)  [unwired: 2 in, 2 out]
                n186 = property on="ParameterPhi" class="NumNb (strict)"() -> ("Value"=w131:dbl)  [unwired: 2 in, 2 out]
                n187 = call "Transmission(Theta) (SubVI).vi"("Theta"=w130, "ParameterA"=w134, "ParameterB"=w133, "ParameterC"=w132, "ParameterPhi"=w131) -> ("Transmission"=w141:dbl)  [unwired: 22 in]
                n188 = property on="Taux transmission calculé" class="NumNb (strict)"("Value"=w141) -> ()  [unwired: 2 in, 2 out]
                n189 = Compound Arithmetic op=OR ("Opérateur arithmétique")(w136, FALSE) -> (w135:bool)
              }
            }
          }
          n190 = Release Queue(queue=w44, error in (no error)=w45) -> (error out=w43:errorcluster)  [unwired: 1 in, 2 out]
          n191 = Merge Errors(w41, w42, w39, w43) -> (w56:errorcluster)
        }
        frame Error {
        }
      }
      "error IO" <- w35
    }
  }
